vi "Mouse click.vi"(8 "error in":errorcluster caption="错误输入（无错误）", 10 "Mouse click":u32(ring)=4 items=["MOVE"=1, "LEFT_DOWN"=2, "lEFT_UP"=4, "RIGHT_DOWN"=8, "RIGHT_UP"=16, "MIDDLE_DOWN"=32, "MIDDLE_UP"=64, "MOUSE_WHEEL"=128, "ABSOLUTE"=32768]) -> (0 "error out":errorcluster)   [LabVIEW 2012]
uses:
  C:/Windows/System32/user32.dll
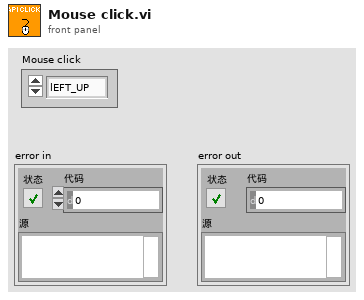
[diagram p1: front panel]
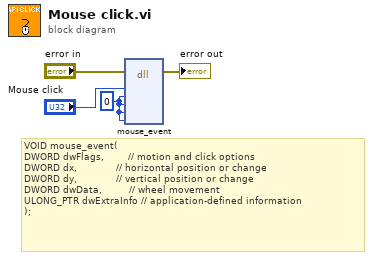
[diagram p0: block diagram]
diagram:
  w4 = u32 0 ("dwExtraInfo")
  # "VOID mouse_event(\nDWORD dwFlags,        // motion and click options\nDWORD dx,             // horizontal position or change\nDWORD dy,             // vertical position or change\nDWORD dwData,         // wheel movement\nULONG_PTR dwExtraInfo // application-defined information\n);"
  n1 = dll-call lib="C:/Windows/System32/user32.dll" fn="mouse_event"(error in="error in", "dwFlags"="Mouse click", "dx"=w4, "dy"=w4, "dwData"=w4, "dwExtraInfo"=w4) -> (error out=→"error out":errorcluster)  [unwired: 8 in, 1 out]
